vi "build_commands.vi"(8 "Refocus_s":u32, 9 "Refocus?":bool, 11 "T1_parameters":T1) -> (3 "instructions_array":T2(array[cluster]))   [LabVIEW 2018]
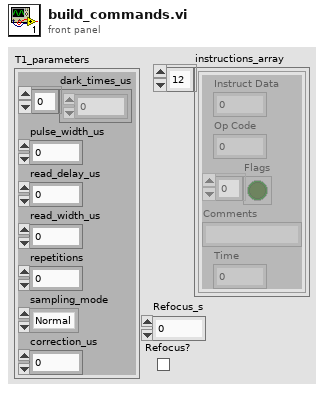
[diagram p1: front panel]
types:
  T1 = cluster{"dark_times_us":dbl[], "pulse_width_us":dbl, "read_delay_us":dbl, "read_width_us":dbl, "repetitions":i32, "sampling_mode":enum16{"Normal", "Sweep"}, "correction_us":dbl}
  T2 = cluster{"Instruct Data":i32, "Op Code":i32, "Flags":bool[], "Comments":string, "Time":dbl}[]
  T3 = cluster{"Instruct Data":i32, "Op Code":i32, "Flags":bool[], "Comments":string, "Time":dbl}
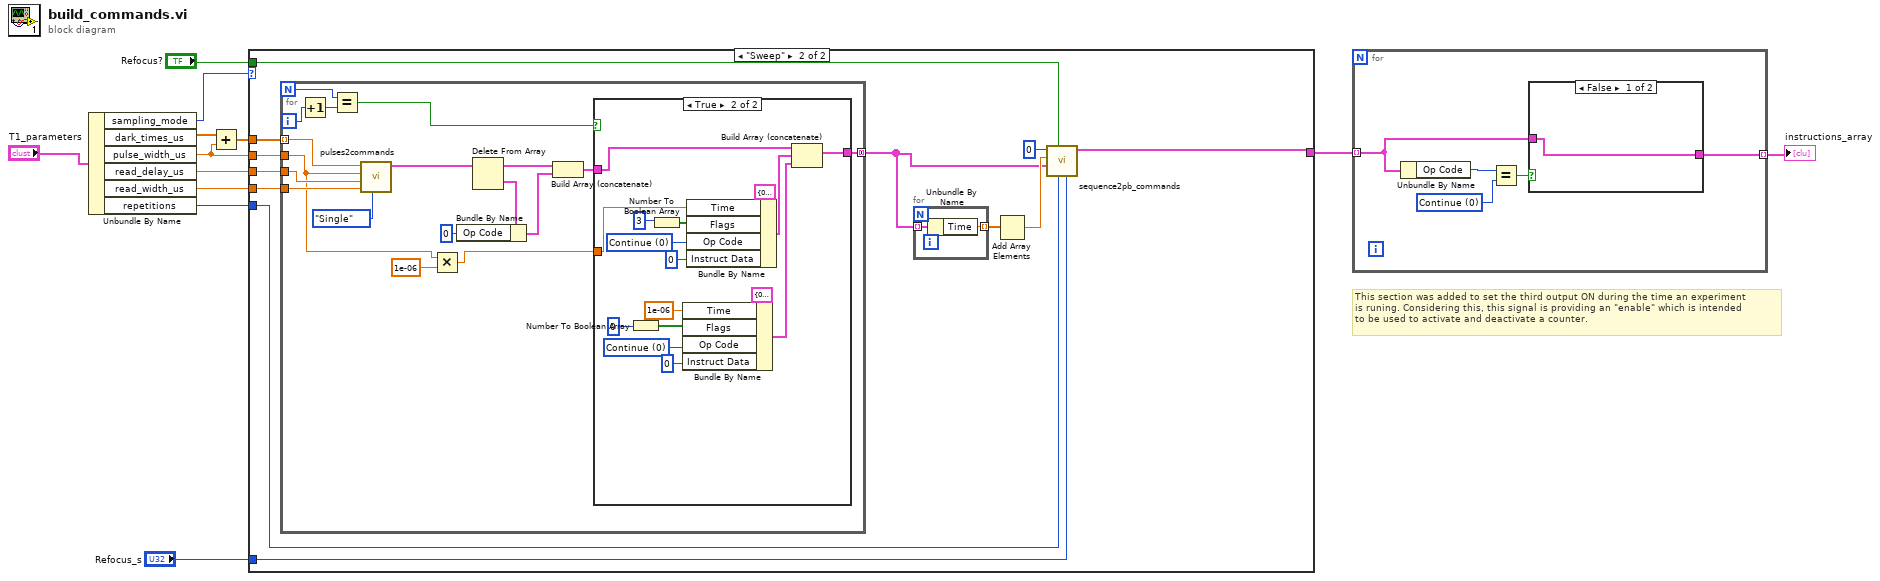
[diagram p0: block diagram]
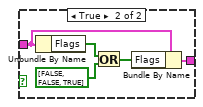
[diagram p2: hidden frame]
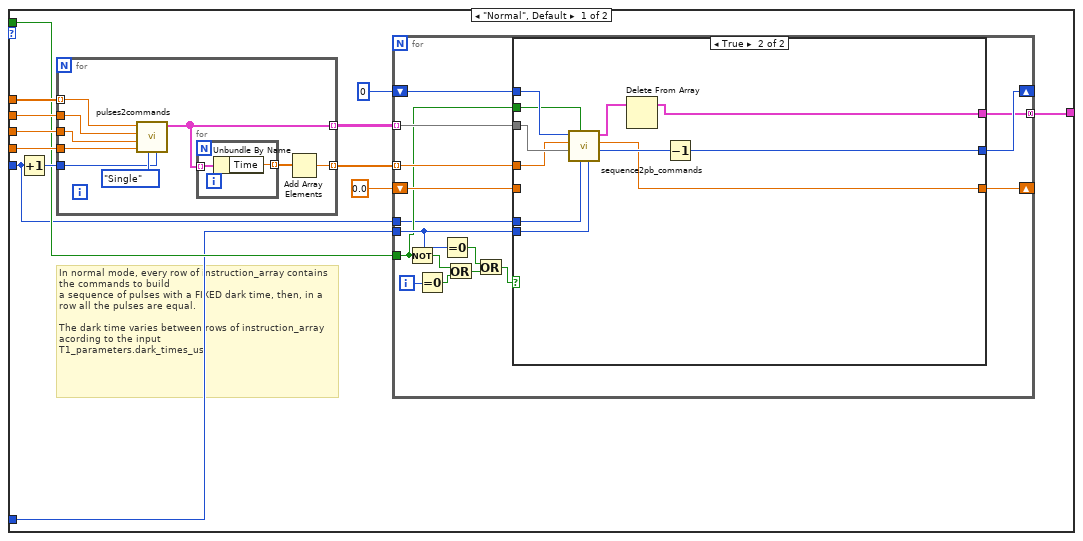
[diagram p3: hidden frame]
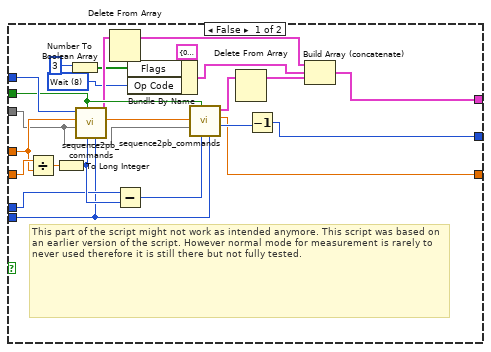
[diagram p4: hidden frame]
diagram:
  # "This section was added to set the third output ON during the time an experiment\nis runing. Considering this, this signal is providing an \"enable\" which is intended\nto be used to activate and deactivate a counter."
  n1 = Unbundle By Name("T1_parameters") -> ("sampling_mode"=w6:enum16{"Normal", "Sweep"}, "dark_times_us"=w7:dbl[], "pulse_width_us"=w9:dbl, "read_delay_us"=w10:dbl, "read_width_us"=w11:dbl, "repetitions"=w12:i32)
  n2 = Add(x=w7, y=w9) -> (x+y=w8:dbl[])
  n3 = case shown="\"Sweep\"" w6 {
    tunnel: w8 -> [w22 w99]
    tunnel: w9 -> [w23 w98]
    tunnel: w10 -> [w24 w97]
    tunnel: w11 -> [w25 w96]
    tunnel: w12 -> [w14 w91]
    tunnel: [w13 w89] -> w1
    tunnel: "Refocus?" -> [w16 w93]
    tunnel: "Refocus_s" -> [w15 w90]
    frame "Normal", Default {
      # "In normal mode, every row of instruction_array contains the commands to build \na sequence of pulses with a FIXED dark time, then, in a row all the pulses are equal.\n\nThe dark time varies between rows of instruction_array acording to the input\nT1_parameters.dark_times_us."
      n4 = Increment(x=w14) -> (x+1=w21:i32)
      n5 = for {
        tunnel: w21 -> [w84]
        tunnel: w25 -> [w83]
        tunnel: w24 -> [w82]
        tunnel: w23 -> [w81]
        tunnel: w22 -> [w80] mode=indexing
        tunnel: [w79] -> w20 mode=indexing
        tunnel: [w77] -> w18 mode=indexing
        n6 = call "pulses2commands.vi"("N_pulses"=w84, "running_mode"=enum16{"Continuous", "Single", "N pulses"}."Single", "read_width_us"=w83, "read_delay_us"=w82, "pulse_width_us"=w81, "pulse_period_us"=w80) -> ("instructions_array"=w79:T2)  [unwired: 4 in, 1 out]
        n7 = for {
          tunnel: w79 -> [w87] mode=indexing
          tunnel: [w86] -> w78 mode=indexing
          n8 = Unbundle By Name(w87) -> ("Time"=w86:dbl)
        }
        n9 = Add Array Elements(numeric array=w78) -> (sum=w77:dbl)
      }
      n10 = for {
        tunnel: w20 -> [w32] mode=indexing
        shift-right: [w27] -> _
        shift-left: 0 -> [w31]
        tunnel: w18 -> [w34] mode=indexing
        shift-right: [w28] -> _
        shift-left: 0.0 -> [w33]
        tunnel: w16 -> [w30]
        tunnel: w15 -> [w36]
        tunnel: w14 -> [w29]
        tunnel: [w26] -> w13 mode=concatenating
        i -> [w41]
        n11 = Not(x=w30) -> (.not. x?=w39:bool)
        n12 = Equal To 0?(x=w41) -> (x = 0?=w40:bool)
        n13 = Equal To 0?(x=w36) -> (x = 0?=w37:bool)
        n14 = Or(x=w39, y=w40) -> (x .or. y?=w38:bool)
        n15 = Or(x=w37, y=w38) -> (x .or. y?=w35:bool)
        n16 = case shown="True" w35 {
          tunnel: w36 -> [w58 w71]
          tunnel: w34 -> [w63 w75]
          tunnel: w33 -> [w65 _]
          tunnel: w32 -> [w57 w76]
          tunnel: w31 -> [w62 w74]
          tunnel: w30 -> [w55 w73]
          tunnel: w29 -> [w59 w72]
          tunnel: [w44 w68] -> w28
          tunnel: [w43 w67] -> w27
          tunnel: [w42 w66] -> w26
          frame False {
            w50 = 8 items=["Continue", "Stop", "Loop", "End Loop", "JSR", "RTS", "Branch", "Long Delay", "Wait"] ("Op Code 2")
            # "This part of the script might not work as intended anymore. This script was based on an earlier version of the script. However normal mode for measurement is rarely to never used therefore it is still there but not fully tested."
            n17 = Divide(x=w65, y=w63) -> (x/y=w64:dbl)
            n18 = To Long Integer(number=w64) -> (32bit integer=w60:i32)
            n19 = Number To Boolean Array(number=3) -> (Boolean array=w51:bool[])
            n20 = call "sequence2pb_commands.vi"("Refocus_s"=w58, "Repetitions"=w60, "Refocus?"=w55, "command_sequence"=w57, "Sequence_length"=w63, "start_command"=w62) -> ("t_remaining"=w56:dbl, "PB_commands"=w54:T2)  [unwired: 3 in, 1 out]
            n21 = Delete From Array(array=w54) -> (array with subset deleted=w47:T2)  [unwired: 2 in, 1 out]
            n22 = Subtract(x=w59, y=w60) -> (x-y=w61:i32)
            n23 = Bundle By Name(cluster=T3 {"Instruct Data"=0, "Op Code"=0, "Flags"=[FALSE, FALSE, FALSE, FALSE, FALSE, FALSE, FALSE, FALSE, FALSE, FALSE, FALSE, FALSE, FALSE, FALSE, FALSE, FALSE, FALSE, FALSE, FALSE, FALSE, FALSE, FALSE, FALSE, FALSE], "Comments"="", "Time"=1e-06} ("PB Instruction"), "Flags"=w51, "Op Code"=w50) -> (w46:T3)
            n24 = call "sequence2pb_commands.vi"("Refocus_s"=w58, "Repetitions"=w61, "Refocus?"=w55, "command_sequence"=w57, "Sequence_length"=w56) -> ("end_command"=w49:i32, "t_remaining"=w44:dbl, "PB_commands"=w48:T2)  [unwired: 4 in]
            n25 = Delete From Array(array=w48) -> (array with subset deleted=w45:T2)  [unwired: 2 in, 1 out]
            n26 = Decrement(x=w49) -> (x-1=w43:i32)
            n27 = Build Array (concatenate)(w47, w46, w45) -> (w42:T2)
          }
          frame True {
            n28 = call "sequence2pb_commands.vi"("Refocus_s"=w71, "Repetitions"=w72, "Refocus?"=w73, "command_sequence"=w76, "Sequence_length"=w75, "start_command"=w74) -> ("end_command"=w69:i32, "t_remaining"=w68:dbl, "PB_commands"=w70:T2)  [unwired: 3 in]
            n29 = Delete From Array(array=w70) -> (array with subset deleted=w66:T2)  [unwired: 2 in, 1 out]
            n30 = Decrement(x=w69) -> (x-1=w67:i32)
          }
        }
      }
    }
    frame "Sweep" {
      n31 = for {
        N -> [w113]
        tunnel: w99 -> [w119] mode=indexing
        tunnel: w98 -> [w104]
        tunnel: w97 -> [w118]
        tunnel: w96 -> [w117]
        tunnel: [w106] -> w88 mode=concatenating
        i -> [w115]
        n32 = Increment(x=w115) -> (x+1=w114:i32)
        n33 = Equal?(x=w113, y=w114) -> (x = y?=w108:bool)
        n34 = call "pulses2commands.vi"("running_mode"=enum16{"Continuous", "Single", "N pulses"}."Single", "read_width_us"=w117, "read_delay_us"=w118, "pulse_width_us"=w104, "pulse_period_us"=w119) -> ("instructions_array"=w107:T2)  [unwired: 5 in, 1 out]
        n35 = Multiply(x=w104, y=1e-06) -> (x*y=w103:dbl)
        n36 = Delete From Array(array=w107) -> (deleted portion=w110:T3, array with subset deleted=w109:T2)  [unwired: 2 in]
        n37 = Bundle By Name(cluster=w110, "Op Code"=0) -> (w111:T3)
        n38 = Build Array (concatenate)(w109, w111) -> (w105:T2)
        n39 = case shown="True" w108 {
          tunnel: [w120 w136] -> w106
          tunnel: w105 -> [w120 w128]
          tunnel: w103 -> [_ w134]
          frame False {
          }
          frame True {
            w126 = 0 items=["Continue", "Stop", "Loop", "End Loop", "JSR", "RTS", "Branch", "Long Delay", "Wait"] ("Op Code 2")
            w131 = 0 items=["Continue", "Stop", "Loop", "End Loop", "JSR", "RTS", "Branch", "Long Delay", "Wait"] ("Op Code 2")
            n40 = Number To Boolean Array(number=0) -> (Boolean array=w124:bool[])
            n41 = Number To Boolean Array(number=3) -> (Boolean array=w132:bool[])
            n42 = Bundle By Name(cluster=T3 {"Instruct Data"=0, "Op Code"=0, "Flags"=[FALSE, FALSE, FALSE, FALSE, FALSE, FALSE, FALSE, FALSE, FALSE, FALSE, FALSE, FALSE, FALSE, FALSE, FALSE, FALSE, FALSE, FALSE, FALSE, FALSE, FALSE, FALSE, FALSE, FALSE], "Comments"="", "Time"=1e-06} ("PB Instruction"), "Time"=1e-06, "Flags"=w124, "Op Code"=w126, "Instruct Data"=0) -> (w121:T3)
            n43 = Bundle By Name(cluster=T3 {"Instruct Data"=0, "Op Code"=0, "Flags"=[FALSE, FALSE, FALSE, FALSE, FALSE, FALSE, FALSE, FALSE, FALSE, FALSE, FALSE, FALSE, FALSE, FALSE, FALSE, FALSE, FALSE, FALSE, FALSE, FALSE, FALSE, FALSE, FALSE, FALSE], "Comments"="", "Time"=1e-06} ("PB Instruction"), "Time"=w134, "Flags"=w132, "Op Code"=w131, "Instruct Data"=0) -> (w129:T3)
            n44 = Build Array (concatenate)(w128, w129, w121) -> (w136:T2)
          }
        }
      }
      n45 = for {
        tunnel: w88 -> [w101] mode=indexing
        tunnel: [w100] -> w95 mode=indexing
        n46 = Unbundle By Name(w101) -> ("Time"=w100:dbl)
      }
      n47 = Add Array Elements(numeric array=w95) -> (sum=w94:dbl)
      n48 = call "sequence2pb_commands.vi"("Refocus_s"=w90, "Repetitions"=w91, "Refocus?"=w93, "command_sequence"=w88, "Sequence_length"=w94, "start_command"=0) -> ("PB_commands"=w89:T2)  [unwired: 3 in, 2 out]
    }
  }
  n49 = for {
    tunnel: w1 -> [w141] mode=indexing
    tunnel: [w140] -> w4 mode=indexing
    w138 = 0 items=["Continue", "Stop", "Loop", "End Loop", "JSR", "RTS", "Branch", "Long Delay", "Wait"] ("Op Code")
    n50 = Unbundle By Name(w141) -> ("Op Code"=w139:i32)
    n51 = Equal?(x=w139, y=w138) -> (x = y?=w137:bool)
    n52 = case shown="False" w137 {
      tunnel: w141 -> [w142 w145]
      tunnel: [w142 w143] -> w140
      frame False {
      }
      frame True {
        n53 = Unbundle By Name(w145) -> ("Flags"=w147:bool[])
        n54 = Or(x=w147, y=bool[] [FALSE, FALSE, TRUE] ("Flags")) -> (x .or. y?=w144:bool[])
        n55 = Bundle By Name(cluster=w145, "Flags"=w144) -> (w143:T3)
      }
    }
  }
  "instructions_array" <- w4
